vi "RS_SMBV100A_DrLL_ESR_check.vi"(4 "Driver Name":string, 6 "Error Code":i32, 7 "Error Query":string, 8 "Error In":errorcluster, 11 "DriverConnect in":T1={"InterfaceType"=enum."VISA", "OpenedSession"="", "InterfaceSettings"={"Interface"=enum."RS232", "EOS 4 read"=enum."LF (\\n)", "EOS 4 write"=enum."LF (\\n)", "TMO, ms"=10000, "Sett"=variant(cluster{"Baud Rate":u32, "Data Bits":u16, "Parity":u16, "Stop Bits":u16, "Flow Control":u16, "Eho":bool} {"Baud Rate"=75, "Data Bits"=0, "Parity"=0, "Stop Bits"=0, "Flow Control"=0, "Eho"=FALSE})}}) -> (0 "Error Out":errorcluster, 3 "DriverConnect out":T1={"InterfaceType"=enum."VISA", "OpenedSession"="", "InterfaceSettings"={"Interface"=enum."RS232", "EOS 4 read"=enum."LF (\\n)", "EOS 4 write"=enum."LF (\\n)", "TMO, ms"=10000, "Sett"=variant(cluster{"Baud Rate":u32, "Data Bits":u16, "Parity":u16, "Stop Bits":u16, "Flow Control":u16, "Eho":bool} {"Baud Rate"=75, "Data Bits"=0, "Parity"=0, "Stop Bits"=0, "Flow Control"=0, "Eho"=FALSE})}})   [LabVIEW 2018]
uses:
  MOKO_LabViewLibrary/MokoLowLevel/MokoLowLovelControl/MLLC_ConnectCluster.ctl
  MOKO_LabViewLibrary/MokoLowLevel/MokoLowLovelControl/MLLC_InterfaceType.ctl
  MOKO_LabViewLibrary/MokoLowLevel/MokoLowLovelControl/MLLC_OpenedSession.ctl
  MOKO_LabViewLibrary/MokoLowLevel/MokoLowLovelControl/MLLC_InterfaceSettings.ctl
  MOKO_LabViewLibrary/MokoLowLevel/MokoLowLovelControl/MLLC_InterfaceKind.ctl
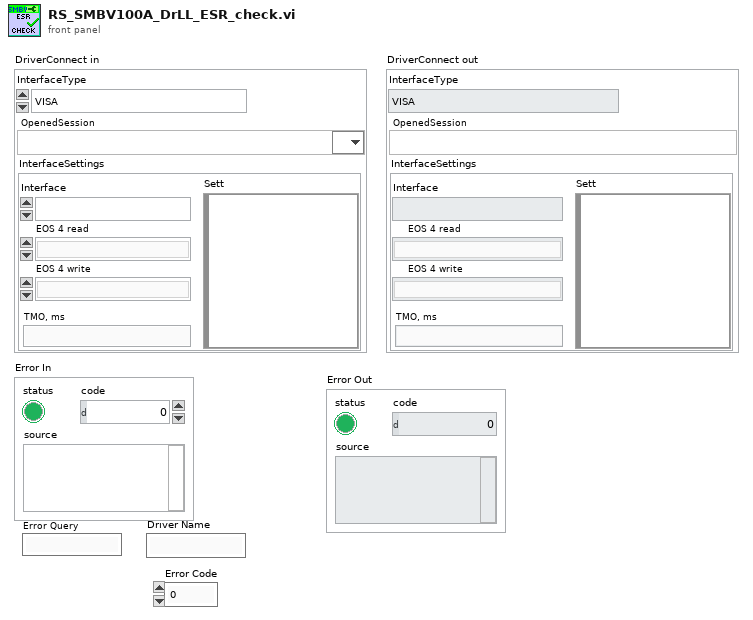
[diagram p1: front panel]
types:
  T1 = typedef "MLLC_ConnectCluster.ctl" = cluster{"InterfaceType":T2, "OpenedSession":T3, "InterfaceSettings":T4}
  T2 = typedef "MLLC_InterfaceType.ctl" = enum16{"VISA", "Prologix USB-GPIB"}
  T3 = typedef "MLLC_OpenedSession.ctl" = refnum<visa-resource-name>
  T4 = typedef "MLLC_InterfaceSettings.ctl" = cluster{"Interface":T5, "EOS 4 read":enum16{"Default (=EOS 4 write)", "CR (\\r)", "LF (\\n)", "None"}, "EOS 4 write":enum16{"CR+LF (\\r\\n)", "CR (\\r)", "LF (\\n)", "None"}, "TMO, ms":i32, "Sett":variant}
  T5 = typedef "MLLC_InterfaceKind.ctl" = enum16{"RS232", "GPIB", "USB", "Ethernet", "another"}
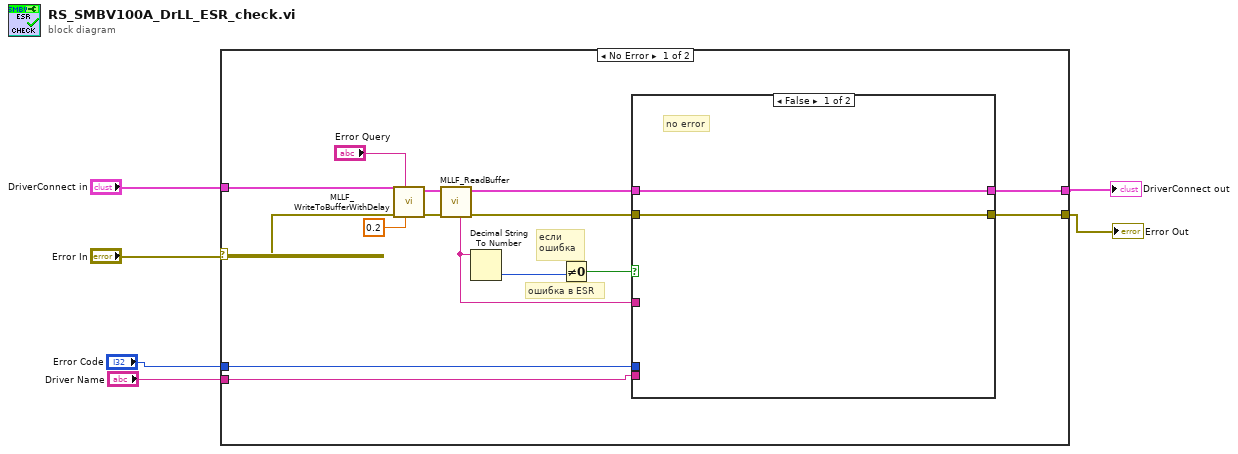
[diagram p0: block diagram]
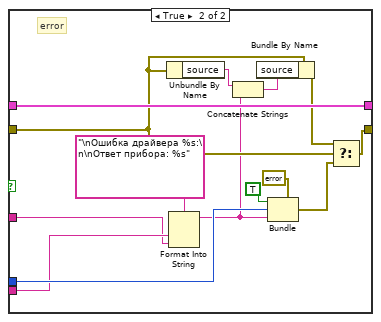
[diagram p2: hidden frame]
diagram:
  n1 = case shown="No Error" "Error In" {
    selector: "Error In" -> [w19 w39]
    tunnel: [w21 w39] -> w3
    tunnel: "DriverConnect in" -> [w20 w38]
    tunnel: [w18 w38] -> w1
    tunnel: "Error Code" -> [w17 _]
    tunnel: "Driver Name" -> [w16 _]
    frame No Error {
      # "ошибка в ESR"
      # "если \nошибка"
      n2 = call "MLLF_WriteToBufferWithDelay.vi"("Delay Time ( 0,05 s)"=0.2 ("Delay Time (s)"), "Command"="Error Query", "Error In"=w19, "DriverConnect in"=w20) -> ("Error Out"=w15:errorcluster, "DriverConnect out"=w14:T1)  [unwired: 6 in]
      n3 = call "MLLF_ReadBuffer.vi"("Error In"=w15, "DriverConnect in"=w14) -> ("Error Out"=w11:errorcluster, "DriverConnect out"=w12:T1, "String"=w9:string)  [unwired: 6 in]
      n4 = Decimal String To Number(string=w9) -> (number=w13:i32)  [unwired: 2 in, 1 out]
      n5 = Not Equal To 0?(x=w13) -> (x != 0?=w10:bool)
      n6 = case shown="False" w10 {
        tunnel: w12 -> [w23 w32]
        tunnel: [w23 w32] -> w18
        tunnel: [w22 w25] -> w21
        tunnel: w11 -> [w22 w31]
        tunnel: w17 -> [_ w34]
        tunnel: w16 -> [_ w33]
        tunnel: w9 -> [_ w24]
        frame False {
          # "no error"
        }
        frame True {
          # "error"
          n7 = Unbundle By Name(w31) -> ("source"=w30:string)
          n8 = Format Into String(format string="\nОшибка драйвера %s:\n\nОтвет прибора: %s", w33, w24) -> (resulting string=w28:string)  [unwired: 2 in, 1 out]
          n9 = Concatenate Strings(w30, w28) -> (w29:string)
          n10 = Bundle By Name(cluster=w31, "source"=w29) -> (w27:errorcluster)
          n11 = Bundle(cluster=errorcluster {"status"=FALSE, "code"=0, "source"=""} ("error out"), "status"=TRUE ("Status"), "code"=w34, "source"=w28) -> (w26:errorcluster)
          n12 = Select(t=w27, s=w31, f=w26) -> (s? t:f=w25:errorcluster)
        }
      }
    }
    frame Error {
    }
  }
  "Error Out" <- w3
  "DriverConnect out" <- w1
